vi "NotifyWithoutData.vi"(8 "error in (no error)":errorcluster, 11 "Communication in":refnum<class "Communication.lvclass">) -> (0 "error out":errorcluster, 2 "Data out":refnum<class "Data.lvclass">, 3 "Communication out":refnum<class "Communication.lvclass">)   [LabVIEW 2023, in "Communication.lvclass"]
doc: "Calls the data class overriding method when the communication method is Notify without data."
uses:
  Communication.lvclass
  Data/Data.lvclass
  Communication.lvclass/Communication.ctl
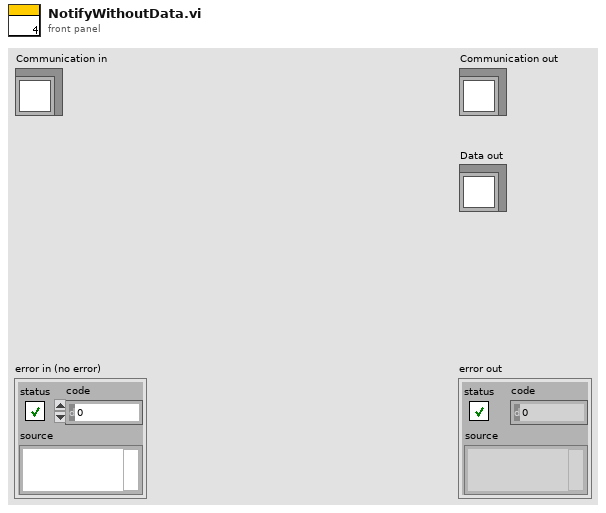
[diagram p1: front panel]
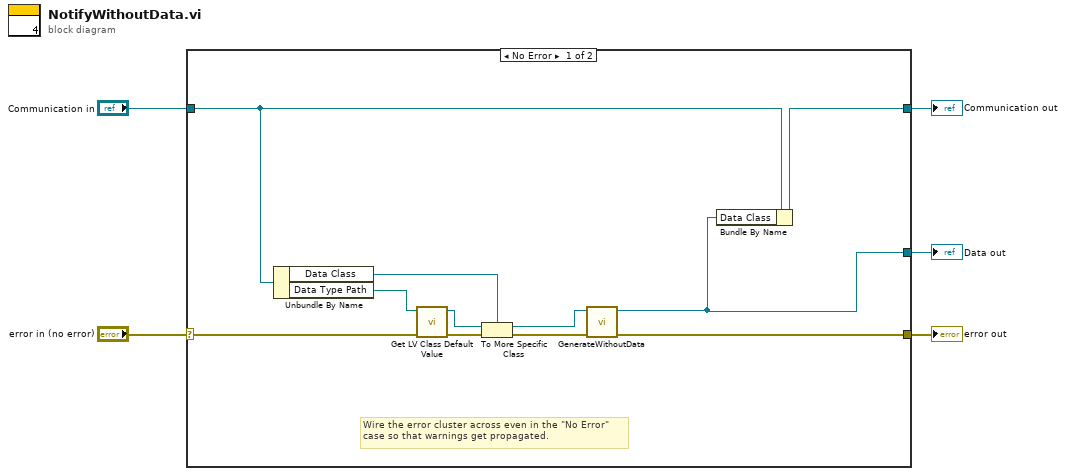
[diagram p0: block diagram]
diagram:
  n1 = case shown="No Error" "error in (no error)" {
    selector: "error in (no error)" -> [w12 w18]
    tunnel: [w6 w18] -> w4
    tunnel: [w10 w17] -> w2
    tunnel: "Communication in" -> [w11 w17]
    tunnel: [w7 _] -> w1
    frame No Error {
      # "Wire the error cluster across even in the \"No Error\"\ncase so that warnings get propagated."
      n2 = Unbundle By Name(w11) -> ("Data Class"=w13:refnum<class "Data.lvclass">, "Data Type Path"=w15:path)
      n3 = call <vilib>:"Get LV Class Default Value.vi"("error in (no error)"=w12, "class path"=w15) -> ("error out"=w16:errorcluster, "object"=w14:refnum<class>)  [unwired: 8 in]
      n4 = To More Specific Class(target class=w13, reference=w14, error in=w16) -> (specific class reference=w9:refnum<class "Data.lvclass">, error out=w8:errorcluster)
      n5 = call-dynamic "GenerateWithoutData.vi"("error in (no error)"=w8, "Data in"=w9) -> ("error out"=w6:errorcluster, "Data out"=w7:refnum<class "Data.lvclass">)  [unwired: 8 in]
      n6 = Bundle By Name(cluster=w11, "Data Class"=w7) -> (w10:refnum<class "Communication.lvclass">)
    }
    frame Error {
    }
  }
  "error out" <- w4
  "Communication out" <- w2
  "Data out" <- w1
